vi "OL Corridor Width.vi"(1 "trial frac":dbl(slide) scale=0.0..1.0, 7 "open loop change positions":string="0,0.25,0.75,1", 12 "open loop values":string="30,15,15,30") -> (8 "ol_wall_array":dbl[](array[numeric]), 10 "col_width":dbl, 15 "Segment Wall Pos (mm)":dbl)   [LabVIEW 2018]
panel:
  out "Segment Fraction":dbl
  out "trial frac":dbl
  # "prev cor pos"
  # "cur cor pos"
  # "prev cor val"
  # "cur cor val"
  # "cor width"
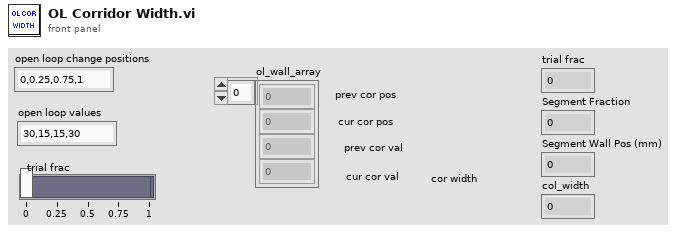
[diagram p1: front panel]
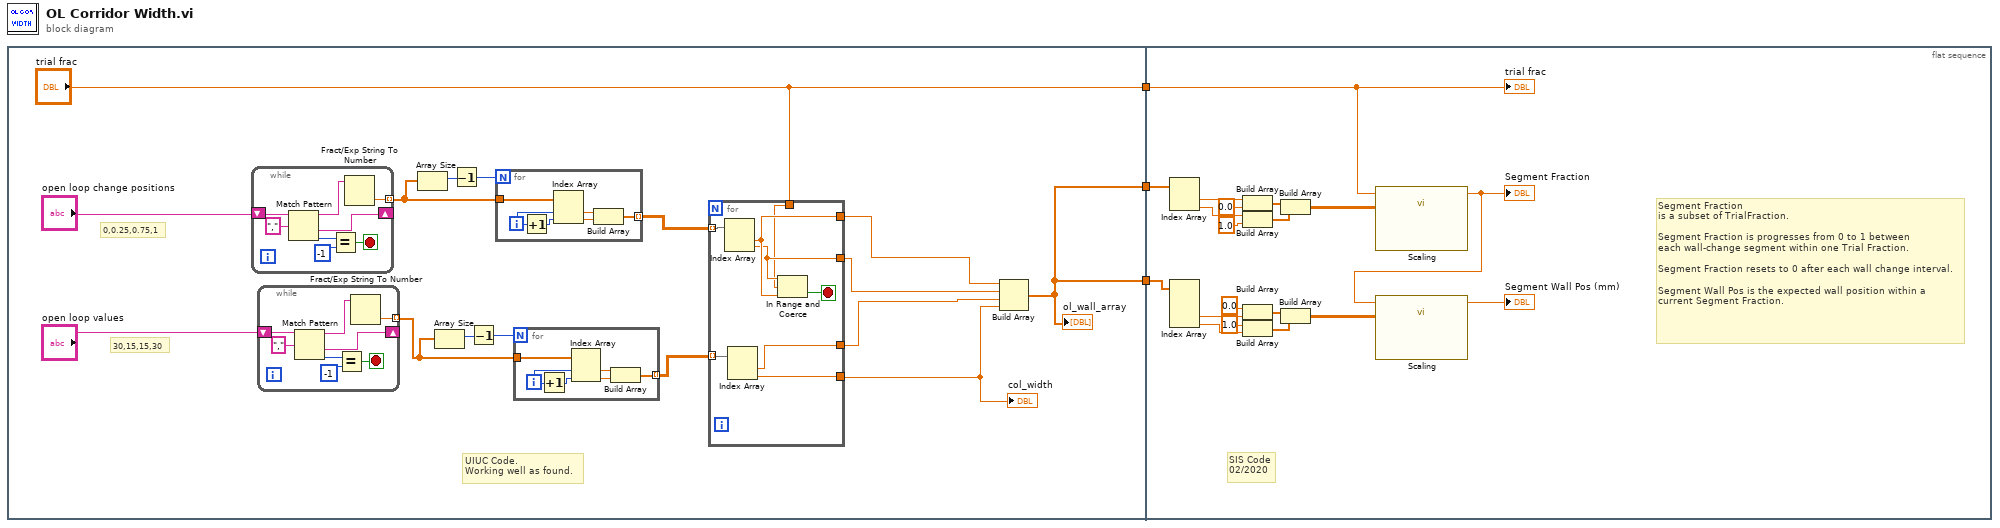
[diagram p0: block diagram]
diagram:
  n1 = flat-sequence {
    tunnel: [w4] -> w3
    tunnel: ["trial frac"] -> w2
    tunnel: [w4] -> w1
    tunnel: w3 -> [w74]
    tunnel: w2 -> [w66]
    tunnel: w1 -> [w63]
    frame #0 {
      # "UIUC Code.\nWorking well as found."
      # "30,15,15,30"
      # "0,0.25,0.75,1"
      n2 = while {
        shift-right: [w48] -> _
        shift-left: "open loop change positions" -> [w54]
        tunnel: [w49] -> w17 mode=indexing
        stop <- w51 stop-if-true
        n3 = Match Pattern(string=w54, regular expression=",") -> (before substring=w50:string, after substring=w48:string, offset past match=w53:i32)  [unwired: 1 in, 1 out]
        n4 = Equal?(x=w53, y=-1) -> (x = y?=w51:bool)
        n5 = Fract/Exp String To Number(string=w50) -> (number=w49:dbl)  [unwired: 3 in, 1 out]
      }
      n6 = while {
        shift-right: [w40] -> _
        shift-left: "open loop values" -> [w46]
        tunnel: [w41] -> w11 mode=indexing
        stop <- w43 stop-if-true
        n7 = Match Pattern(string=w46, regular expression=",") -> (before substring=w42:string, after substring=w40:string, offset past match=w45:i32)  [unwired: 1 in, 1 out]
        n8 = Equal?(x=w45, y=-1) -> (x = y?=w43:bool)
        n9 = Fract/Exp String To Number(string=w42) -> (number=w41:dbl)  [unwired: 3 in, 1 out]
      }
      n10 = Array Size(array=w17) -> (size(s)=w19:i32)
      n11 = Array Size(array=w11) -> (size(s)=w13:i32)
      n12 = Decrement(x=w19) -> (x-1=w18:i32)
      n13 = Decrement(x=w13) -> (x-1=w12:i32)
      n14 = for {
        N: w18 -> [_]
        tunnel: w17 -> [w37]
        tunnel: [w34] -> w16 mode=indexing
        i -> [w38]
        n15 = Increment(x=w38) -> (x+1=w39:i32)
        n16 = Index Array(array=w37, index #1=w38, index #2=w39) -> (element #1=w36:dbl, element #2=w35:dbl)
        n17 = Build Array(w36, w35) -> (w34:dbl[])
      }
      n18 = for {
        N: w12 -> [_]
        tunnel: w11 -> [w23]
        tunnel: [w20] -> w10 mode=indexing
        i -> [w24]
        n19 = Increment(x=w24) -> (x+1=w25:i32)
        n20 = Index Array(array=w23, index #1=w24, index #2=w25) -> (element #1=w22:dbl, element #2=w21:dbl)
        n21 = Build Array(w22, w21) -> (w20:dbl[])
      }
      n22 = for {
        tunnel: w16 -> [w33] mode=indexing
        tunnel: "trial frac" -> [w30]
        tunnel: [w32] -> w9
        tunnel: [w31] -> w8
        tunnel: w10 -> [w29] mode=indexing
        tunnel: [w28] -> w6
        tunnel: [w27] -> w7
        stop <- w26 stop-if-true
        n23 = Index Array(array=w33) -> (element #1=w32:dbl, element #2=w31:dbl)  [unwired: 2 in]
        n24 = Index Array(array=w29) -> (element #1=w27:dbl, element #2=w28:dbl)  [unwired: 2 in]
        n25 = In Range and Coerce(upper limit=w31, x=w30, lower limit=w32) -> (In Range?=w26:bool)  [unwired: 1 out]
      }
      "col_width" <- w6
      n26 = Build Array(w9, w8, w7, w6) -> (w4:dbl[])
      "ol_wall_array" <- w4
    }
    frame #1 {
      # "SIS Code\n02/2020"
      # "Segment Fraction\nis a subset of TrialFraction.\n\nSegment Fraction is progresses from 0 to 1 between\neach wall-change segment within one Trial Fraction.\n\nSegment Fraction resets to 0 after each wall change interval.\n\nSegment Wall Pos is the expected wall position within a \ncurrent Segment Fraction."
      n27 = Index Array(array=w74) -> (element #1=w73:dbl, element #2=w72:dbl)  [unwired: 2 in]
      n28 = Index Array(array=w63) -> (element #3=w60:dbl, element #4=w59:dbl)  [unwired: 4 in, 2 out]
      n29 = Build Array(w73, 0.0 ("element")) -> (w68:dbl[])
      n30 = Build Array(w72, 1.0 ("element")) -> (w69:dbl[])
      n31 = Build Array(0.0 ("element"), w60) -> (w65:dbl[])
      n32 = Build Array(1.0 ("element"), w59) -> (w64:dbl[])
      n33 = Build Array(w68, w69) -> (w67:dbl[][])
      n34 = Build Array(w65, w64) -> (w58:dbl[][])
      n35 = call "Scaling.vi"("Interpolation Points"=w67, "Input"=w66) -> ("Output"=w57:dbl)  [unwired: 8 in, 1 out]
      "Segment Fraction" <- w57
      n36 = call "Scaling.vi"("Interpolation Points"=w58, "Input"=w57) -> ("Output"=→"Segment Wall Pos (mm)":dbl)  [unwired: 8 in, 1 out]
      "trial frac" <- w66
    }
  }
